vi "TDT-Get Ticks.vi"(0 "Data":T1={"TTankX"=refnum, "TDevAccX"=refnum, "LastTime"=0.0, "error"={"status"=FALSE, "code"=0, "source"=""}, "Block Name"="", "Circuit Tag"="", "Tank Name"="", "NumTicks"=0, "LastTick"=0.0, "Idle?"=FALSE, "Wait (ms)"=1000, "LastArtf"=0.0, "LastTosc"=0.0}, 5 "T2":dbl, 7 "Max Read":i32=1000, 11 "error in (no error)":errorcluster) -> (4 "Got 'em all":bool, 6 "Number of Ticks":i32, 8 "Tick times":dbl[][](array[numeric]), 15 "error out":errorcluster)   [LabVIEW 2015]
uses:
  TDT Interface Data.ctl
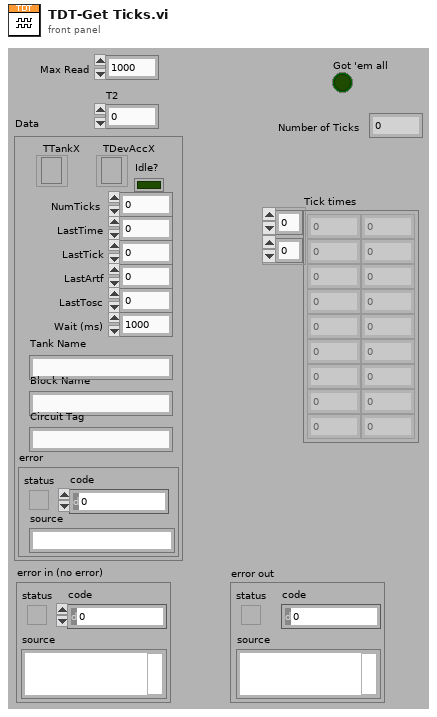
[diagram p1: front panel]
types:
  T1 = typedef "TDT Interface Data.ctl" = cluster{"TTankX":refnum<k7>, "TDevAccX":refnum<k7>, "LastTime":dbl, "error":errorcluster, "Block Name":string, "Circuit Tag":string, "Tank Name":string, "NumTicks":i32, "LastTick":dbl, "Idle?":bool, "Wait (ms)":u32, "LastArtf":dbl, "LastTosc":dbl}
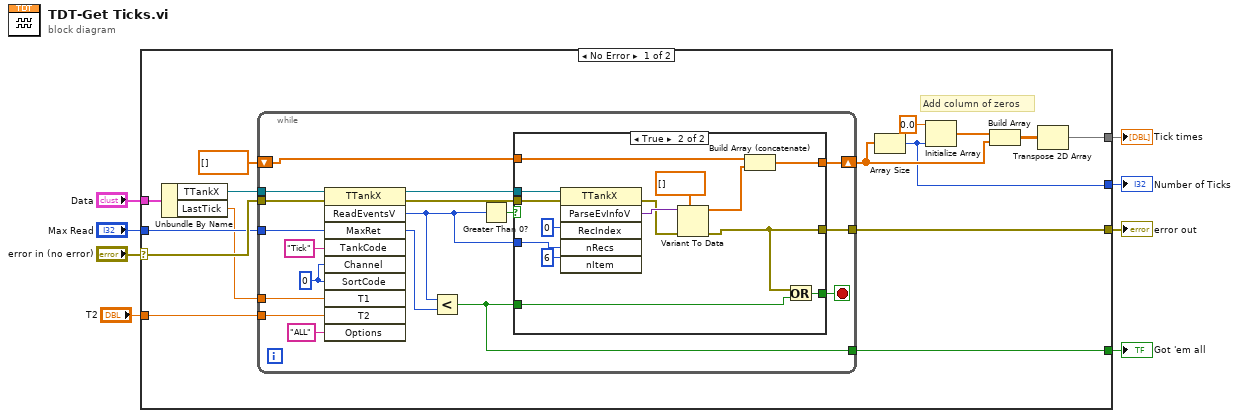
[diagram p0: block diagram]
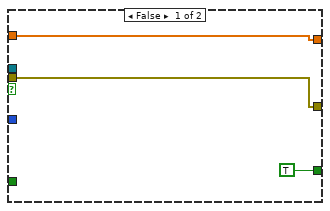
[diagram p2: hidden frame]
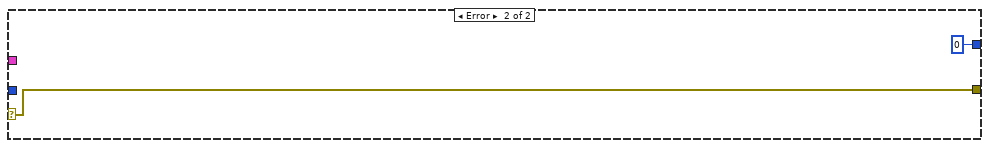
[diagram p3: hidden frame]
diagram:
  n1 = case shown="No Error" "error in (no error)" {
    selector: "error in (no error)" -> [w21 w60]
    tunnel: "Data" -> [w23 _]
    tunnel: "Max Read" -> [w20 _]
    tunnel: [w17 w60] -> w5
    tunnel: [w12 _] -> w4
    tunnel: [w11 0] -> w3
    tunnel: "T2" -> [w10 _]
    tunnel: [w9 _] -> w1
    frame No Error {
      # "Add column of zeros"
      n2 = Unbundle By Name(w23) -> ("TTankX"=w22:refnum<k7>, "LastTick"=w19:dbl)
      n3 = while {
        tunnel: w22 -> [w41]
        tunnel: w21 -> [w40]
        tunnel: w20 -> [w39]
        tunnel: w19 -> [w25]
        shift-right: [w31] -> w14
        shift-left: dbl[] [] -> [w30]
        tunnel: [w29] -> w17
        tunnel: w10 -> [w24]
        tunnel: [w26] -> w9
        stop <- w34 stop-if-true
        w37 = 0 ("Channel")
        n4 = invoke class="TTankX" method="ReadEventsV"(reference=w41, error in=w40, "MaxRet"=w39, "TankCode"="Tick", "Channel"=w37, "SortCode"=w37, "T1"=w25, "T2"=w24, "Options"="ALL") -> (reference out=w33:refnum<k7>, error out=w32:errorcluster, "ReadEventsV"=w27:i32, "MaxRet"=w35:i32)  [unwired: 1 in, 6 out]
        n5 = Less?(x=w27, y=w35) -> (x < y?=w26:bool)
        n6 = Greater Than 0?(x=w27) -> (x > 0?=w28:bool)
        n7 = case shown="True" w28 {
          tunnel: [TRUE w58] -> w34
          tunnel: w26 -> [_ w57]
          tunnel: w33 -> [_ w56]
          tunnel: w32 -> [w43 w55]
          tunnel: w27 -> [_ w53]
          tunnel: [w44 w47] -> w31
          tunnel: w30 -> [w44 w46]
          tunnel: [w43 w45] -> w29
          frame False {
          }
          frame True {
            n8 = invoke class="TTankX" method="ParseEvInfoV"(reference=w56, error in=w55, "RecIndex"=0, "nRecs"=w53, "nItem"=6) -> (error out=w49:errorcluster, "ParseEvInfoV"=w51:variant)  [unwired: 1 in, 4 out]
            n9 = Variant To Data(error in=w49, type=dbl[] [], Variant=w51) -> (data=w48:dbl[], error out=w45:errorcluster)
            n10 = Build Array (concatenate)(w46, w48) -> (w47:dbl[])
            n11 = Or(x=w45, y=w57) -> (x .or. y?=w58:bool)
          }
        }
      }
      n12 = Array Size(array=w14) -> (size(s)=w11:i32)
      n13 = Initialize Array(0.0 ("element"), w11) -> (w15:dbl[])
      n14 = Build Array(w15, w14) -> (w13:dbl[][])
      n15 = Transpose 2D Array(2D array=w13) -> (transposed array=w12:dbl[][])
    }
    frame Error {
    }
  }
  "Tick times" <- w4
  "error out" <- w5
  "Number of Ticks" <- w3
  "Got 'em all" <- w1
